vi "Configure Extended Network Connection.vi"(5 "Interval (20s)":i32=20, 6 "User Agent (WattsUp.NET)":string="WattsUp.NET", 7 "Port (80)":i32=80, 8 "error in (no error)":errorcluster, 9 "File (/remote/netlog.php)":string="/remote/netlog.php", 10 "Host (data.wattsupmeters.com)":string="data.wattsupmeters.com", 11 "VISA resource name":refnum<visa-resource-name>) -> (0 "error out":errorcluster, 3 "VISA resource name out":refnum<visa-resource-name>)   [LabVIEW 2013, in "Watts Up Series.lvlib"]
doc: "Configure and set extended network settings for the Watts Up .Net device. The default values are for use with Watts Up online terminal, found at <b>https://data.wattsupmeters.com/login.php</b>.\n\nIf you intend to use the online service, please do not change these settings. If you would like to use the Watts Up .Net for use with your own server, then change the configuration to match your server's information."
uses:
  <instrlib>/Watts Up Series/Watts Up Series.lvlib
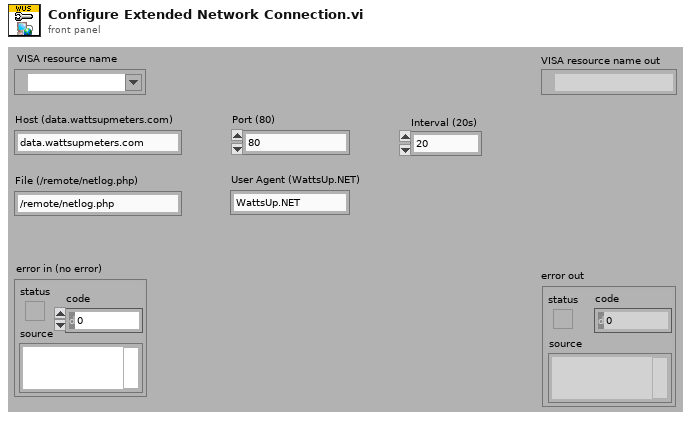
[diagram p1: front panel]
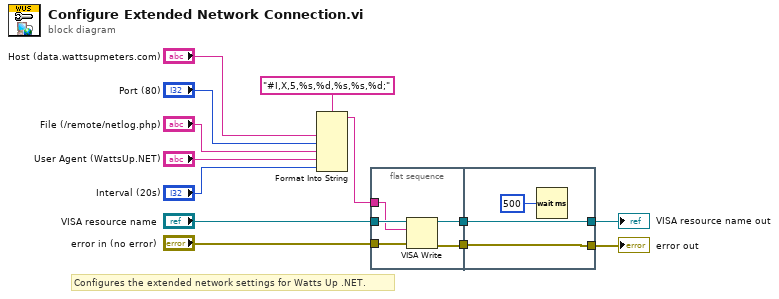
[diagram p0: block diagram]
diagram:
  # "Configures the extended network settings for Watts Up .NET."
  n1 = Format Into String(format string="#I,X,5,%s,%d,%s,%s,%d;", "Host (data.wattsupmeters.com)", "Port (80)", "File (/remote/netlog.php)", "User Agent (WattsUp.NET)", "Interval (20s)") -> (resulting string=w1:string)  [unwired: 2 in, 1 out]
  n2 = flat-sequence {
    tunnel: "VISA resource name" -> [w18]
    tunnel: "error in (no error)" -> [w15]
    tunnel: [w17] -> w3
    tunnel: [w16] -> w2
    tunnel: w1 -> [w14]
    tunnel: [w20] -> w5
    tunnel: [w21] -> w6
    tunnel: w3 -> [w21]
    tunnel: w2 -> [w20]
    frame #0 {
      n3 = VISA Write(VISA resource name=w18, write buffer=w14, error in (no error)=w15) -> (VISA resource name out=w17:refnum<visa-resource-name>, error out=w16:errorcluster)  [unwired: 1 out]
    }
    frame #1 {
      n4 = Wait (ms)(milliseconds to wait=u32 500) -> ()  [unwired: 1 out]
    }
  }
  "VISA resource name out" <- w6
  "error out" <- w5
